vi "GetItemInformationFromProjects.vi"(8 "error in (no error)":errorcluster, 11 "SolutionBuilder in":refnum<class "SolutionBuilder.lvclass">) -> (0 "error out":errorcluster, 3 "SolutionBuilder out":refnum<class "SolutionBuilder.lvclass">)   [LabVIEW 2020, in "SolutionBuilder.lvlib" / "SolutionBuilder.lvclass"]
uses:
  SolutionBuilder.lvclass
  SolutionBuilder.lvclass/SolutionBuilder.ctl
  2db24307-6a08-44b6-ad1c-d8e15639a4a8.vi
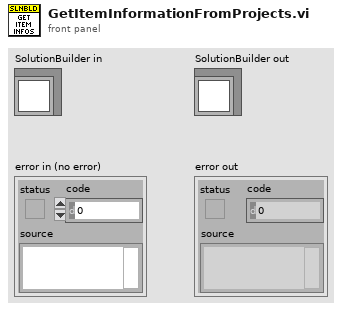
[diagram p1: front panel]
types:
  T1 = typedef "SolutionBuilder.lvlib/SolutionBuilder.lvclass/ItemInfo.ctl" = map{string, T2}
  T2 = typedef "SolutionBuilder.lvlib/SolutionBuilder.lvclass/ProjectInfo.ctl" = cluster{"Deps":set{string}, "FileInfo":T3}
  T3 = typedef "SolutionBuilder.lvlib/SolutionBuilder.lvclass/FileInfo.ctl" = cluster{"Library ref":refnum<vi>, "Target path":path, "Source name":string, "Build spec name":string}
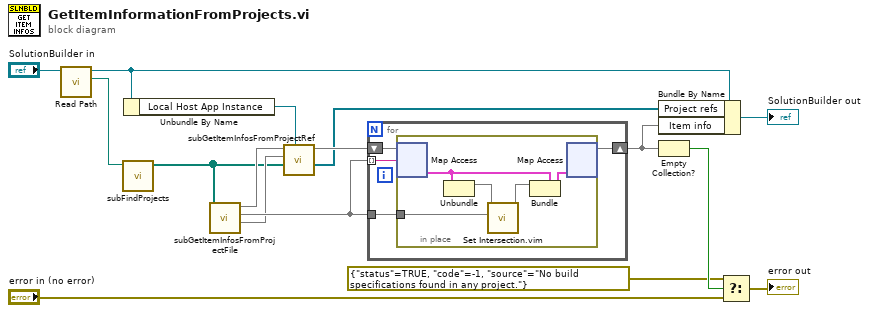
[diagram p0: block diagram]
diagram:
  n1 = call-dynamic "Read Path.vi"("SolutionBuilder in"="SolutionBuilder in") -> ("Path"=w14:path, "SolutionBuilder out"=w9:refnum<class "SolutionBuilder.lvclass">)  [unwired: 9 in]
  n2 = call "subFindProjects.vi"("Path"=w14) -> ("All Files in Dir"=w8:path[])  [unwired: 10 in]
  n3 = Unbundle By Name(w9) -> ("Local Host App Instance"=w7:refnum<vi>)
  n4 = call "subGetItemInfosFromProjectFile.vi"("All Files in Dir"=w8) -> ("Source dist"=w10:map{string, set{string}}, "TargetFile name"=w13:set{string}, "TargetFile info"=w12:T1)  [unwired: 8 in]
  n5 = call "subGetItemInfosFromProjectRef.vi"("Local Host App Instance"=w7, "All Files in Dir"=w8, "Source dist"=w10, "TargetFile info in"=w12) -> ("Project refs"=w6:refnum<vi>[], "TargetFile info"=w11:T1)  [unwired: 6 in]
  n6 = for {
    tunnel: w13 -> [w20]
    tunnel: w13 -> [w18] mode=indexing
    shift-right: [w17] -> w5
    shift-left: w11 -> [w19]
    n7 = in-place {
      in-place-border: w20 -> [w24]
      n8 = in-place-map #1(w19, w18) -> (w21:T2)  [unwired: 1 in, 1 out]
      n9 = Unbundle(w21) -> ("Deps"=w25:set{string})  [unwired: 1 out]
      n10 = call "Set Intersection.vim"("set 2"=w24, "set 1"=w25) -> ("intersection"=w23:set{string})  [unwired: 9 in]
      n11 = Bundle(cluster=w21, "Deps"=w23) -> (w22:T2)  [unwired: 1 in]
      n12 = in-place-map #1(w22) -> (w17:T1)  [unwired: 1 in, 2 out]
    }
  }
  n13 = Bundle By Name(cluster=w9, "Project refs"=w6, "Item info"=w5) -> (→"SolutionBuilder out":refnum<class "SolutionBuilder.lvclass">)
  n14 = Empty Collection?(1:w5) -> (0:w4:bool)
  n15 = Select(t=errorcluster {"status"=TRUE, "code"=-1, "source"="No build specifications found in any project."}, s=w4, f="error in (no error)") -> (s? t:f=→"error out":errorcluster)
